vi "SubVI_Tree_Loaded.vi"(8 "error in (no error)":errorcluster, 10 "Group/Timestrings Cls":cluster{string, string[]}[](array[cluster]), 11 "Tree":refnum<vi>) -> (0 "error out":errorcluster)   [LabVIEW 2018]
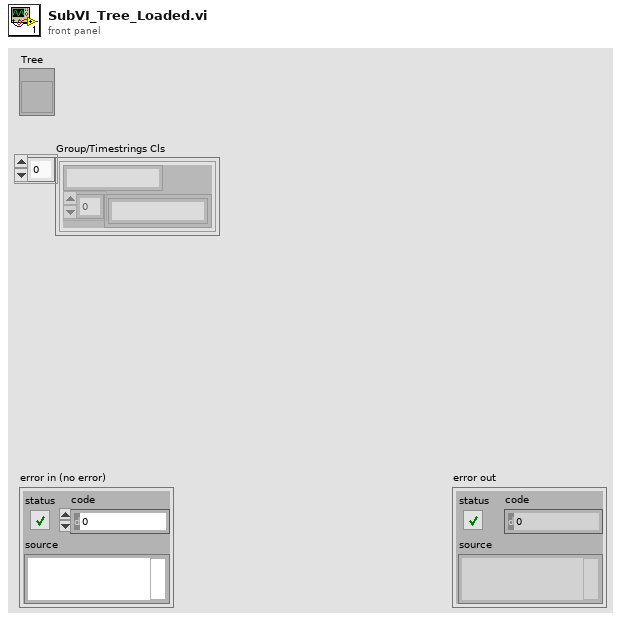
[diagram p1: front panel]
types:
  T1 = cluster{"Left Cell String":string, "Child Text":string[], "Child Tag":string, "Item Indent":i32, "Child Only?":bool, "Glyph Index":i32}
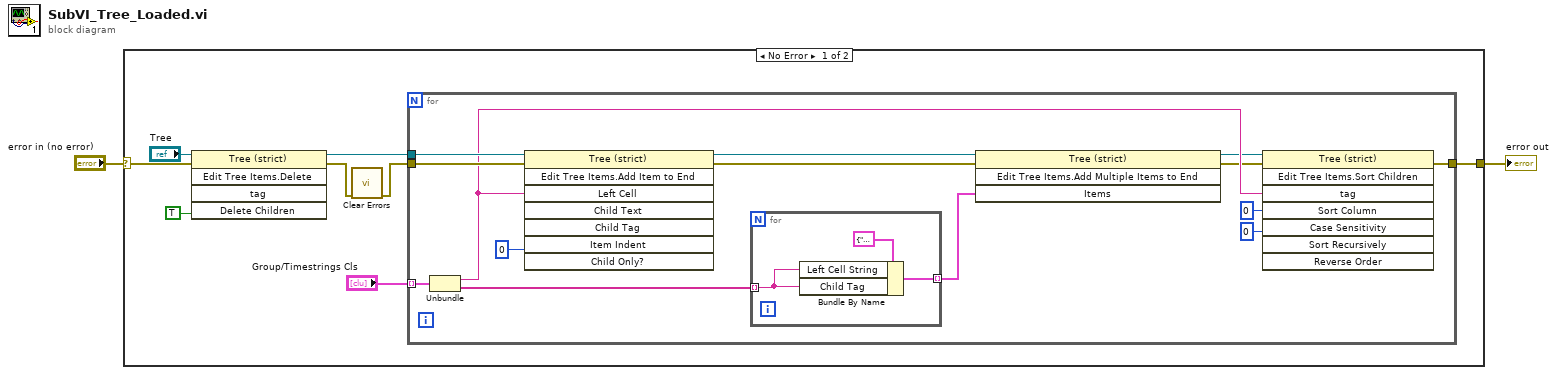
[diagram p0: block diagram]
diagram:
  n1 = case shown="No Error" "error in (no error)" {
    selector: "error in (no error)" -> [w4 w28]
    tunnel: [w5 w28] -> w2
    frame No Error {
      n2 = invoke class="Tree (strict)" method="Edit Tree Items.Delete"(reference="Tree", error in=w4, "Delete Children"=TRUE ("Delete Children?")) -> (reference out=w3:refnum<vi>, error out=w7:errorcluster)  [unwired: 2 in, 3 out]
      n3 = call <vilib>:"Clear Errors.vi"("error in (no error)"=w7) -> ("error out"=w6:errorcluster)  [unwired: 5 in, 1 out]
      n4 = for {
        tunnel: w3 -> [w22]
        tunnel: w6 -> [w23]
        tunnel: "Group/Timestrings Cls" -> [w24] mode=indexing
        tunnel: [w17] -> w5
        n5 = Unbundle(w24) -> (w20:string, w16:string[])
        n6 = invoke class="Tree (strict)" method="Edit Tree Items.Add Item to End"(reference=w22, error in=w23, "Left Cell"=w20, "Item Indent"=0 ("New Item Indentation")) -> (reference out=w15:refnum<vi>, error out=w14:errorcluster)  [unwired: 4 in, 6 out]
        n7 = for {
          tunnel: w16 -> [w26] mode=indexing
          tunnel: [w25] -> w11 mode=indexing
          n8 = Bundle By Name(cluster=T1 {"Left Cell String"="", "Child Text"=[], "Child Tag"="", "Item Indent"=1, "Child Only?"=TRUE, "Glyph Index"=0} ("Item"), "Left Cell String"=w26, "Child Tag"=w26) -> (w25:T1)
        }
        n9 = invoke class="Tree (strict)" method="Edit Tree Items.Add Multiple Items to End"(reference=w15, error in=w14, "Items"=w11) -> (reference out=w13:refnum<vi>, error out=w12:errorcluster)  [unwired: 1 in, 2 out]
        n10 = invoke class="Tree (strict)" method="Edit Tree Items.Sort Children"(reference=w13, error in=w12, "tag"=w20, "Sort Column"=0, "Case Sensitivity"=0) -> (error out=w17:errorcluster)  [unwired: 3 in, 7 out]
      }
    }
    frame Error {
    }
  }
  "error out" <- w2
